vi "Clean_Scanned_Indices.vi"(11 "Rows in":T1[](array[typedef])) -> (3 "Rows out":T1[](array[typedef]))   [LabVIEW 2016]
doc: "<B>Description:</B> Works through a Scanned Index array and removes elements from the top until the first element is a Not Scanned and the second and Third element are Scanned.\n\n<B>Date:</B> 03/2019\n<B>Author:</B> Luke Jarocki, Choose Movement Consulting, LLC"
uses:
  Controls/Scan_Values.ctl
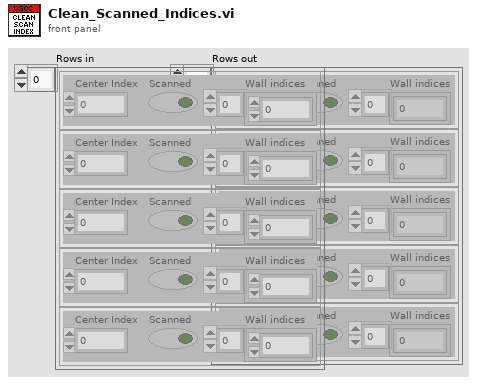
[diagram p1: front panel]
types:
  T1 = typedef "Scan_Values.ctl" = cluster{"Center Index":i32, "Scanned":bool, "Wall indices":i32[]}
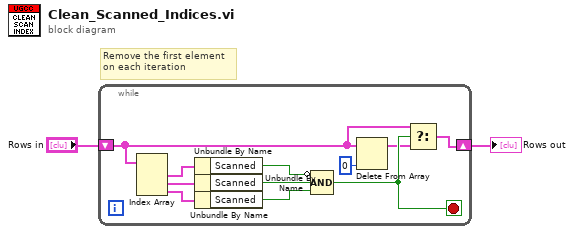
[diagram p0: block diagram]
diagram:
  # "Remove the first element\non each iteration"
  n1 = while {
    shift-right: [w3] -> w2
    shift-left: "Rows in" -> [w4]
    stop <- w6 stop-if-true
    n2 = Index Array(array=w4) -> (element #1=w13:T1, element #2=w12:T1, element #3=w11:T1)  [unwired: 3 in]
    n3 = Unbundle By Name(w13) -> ("Scanned"=w10:bool)
    n4 = Unbundle By Name(w12) -> ("Scanned"=w9:bool)
    n5 = Unbundle By Name(w11) -> ("Scanned"=w8:bool)
    n6 = Compound Arithmetic op=AND(invert w10, w9, w8) -> (w6:bool)
    n7 = Delete From Array(array=w4, index=0) -> (array with subset deleted=w5:T1[])  [unwired: 1 in, 1 out]
    n8 = Select(t=w4, s=w6, f=w5) -> (s? t:f=w3:T1[])
  }
  "Rows out" <- w2
